vi "Export Routines.vi"(8 "error in (no error)":errorcluster, 10 "GUID":string, 11 "Section Ref in":T4 format="%.0x") -> (0 "error out":errorcluster, 1 "Routines":T1 {"Stop.Resp"."Signals"."Byte Order" items=["Little Endian", "Big Endian"]; "Stop.Resp"."Signals"."Data Type" items=["Signed", "Unsigned", "IEEE Float"]; "Stop.Cmd"."Signals"."Byte Order" items=["Little Endian", "Big Endian"]; "Stop.Cmd"."Signals"."Data Type" items=["Signed", "Unsigned", "IEEE Float"]; "Request.Resp"."Signals"."Byte Order" items=["Little Endian", "Big Endian"]; "Request.Resp"."Signals"."Data Type" items=["Signed", "Unsigned", "IEEE Float"]; "Request.Cmd"."Signals"."Byte Order" items=["Little Endian", "Big Endian"]; "Request.Cmd"."Signals"."Data Type" items=["Signed", "Unsigned", "IEEE Float"]; "Start.Resp"."Signals"."Byte Order" items=["Little Endian", "Big Endian"]; "Start.Resp"."Signals"."Data Type" items=["Signed", "Unsigned", "IEEE Float"]; "Start.Cmd"."Signals"."Byte Order" items=["Little Endian", "Big Endian"]; "Start.Cmd"."Signals"."Data Type" items=["Signed", "Unsigned", "IEEE Float"]}, 2 "Routine Refs":T5 {"Stop.Resp"."Signal Refs" format="%.0x"; "Stop.Cmd"."Signal Refs" format="%.0x"; "Status.Resp"."Signal Refs" format="%.0x"; "Status.Cmd"."Signal Refs" format="%.0x"; "Start.Resp"."Signal Refs" format="%.0x"; "Start.Cmd"."Signal Refs" format="%.0x"}, 3 "Section Ref out":T4 format="%.0x")   [LabVIEW 2015, in "Diagnostics Addon System Explorer.lvlib"]
uses:
  Diagnostics Addon System Explorer.lvlib
  <vilib>/NI Veristand/Custom Device API/Custom Device Item Ref.ctl
  Types/Routine VS References.ctl
  Types/Frame Signal VS References.ctl
  Shared/Types/Common Routines.ctl
  Shared/Types/Common Frame Parameters.ctl
  Shared/Types/Signal Parameters.ctl
  Types/FG Action.ctl
  Signal Parameters FG.vi
  <vilib>/NI Veristand/Custom Device API/NI VeriStand - Get Custom Device Channel Data.vi
  <vilib>/NI Veristand/Custom Device API/NI VeriStand - Get Item Description.vi
  <vilib>/NI Veristand/Custom Device API/NI VeriStand - Get Item Property.vi
  <vilib>/NI Veristand/Custom Device API/Get Item Property (String).vi
  <vilib>/NI Veristand/Custom Device API/Get Item Property (Double).vi
  <vilib>/NI Veristand/Custom Device API/Get Item Property (U32).vi
  <vilib>/NI Veristand/Custom Device API/NI VeriStand - Set Item Property.vi
  <vilib>/NI Veristand/Custom Device API/Set Item Property (String).vi
  <vilib>/NI Veristand/Custom Device API/Set Item Property (Double).vi
  <vilib>/NI Veristand/Custom Device API/Set Item Property (U32).vi
  Shared/SubVIs/GUID Lookup.vi
  <vilib>/NI Veristand/Custom Device Tools/Custom Device Utility Library/NI VeriStand - Search for Item by GUID.vi
  <vilib>/NI Veristand/Custom Device Tools/Custom Device Utility Library/Custom Device Utility Library.lvlib
  <vilib>/NI Veristand/Custom Device API/Custom Device API.lvlib
  Shared/Diagnostics Addon Shared.lvlib
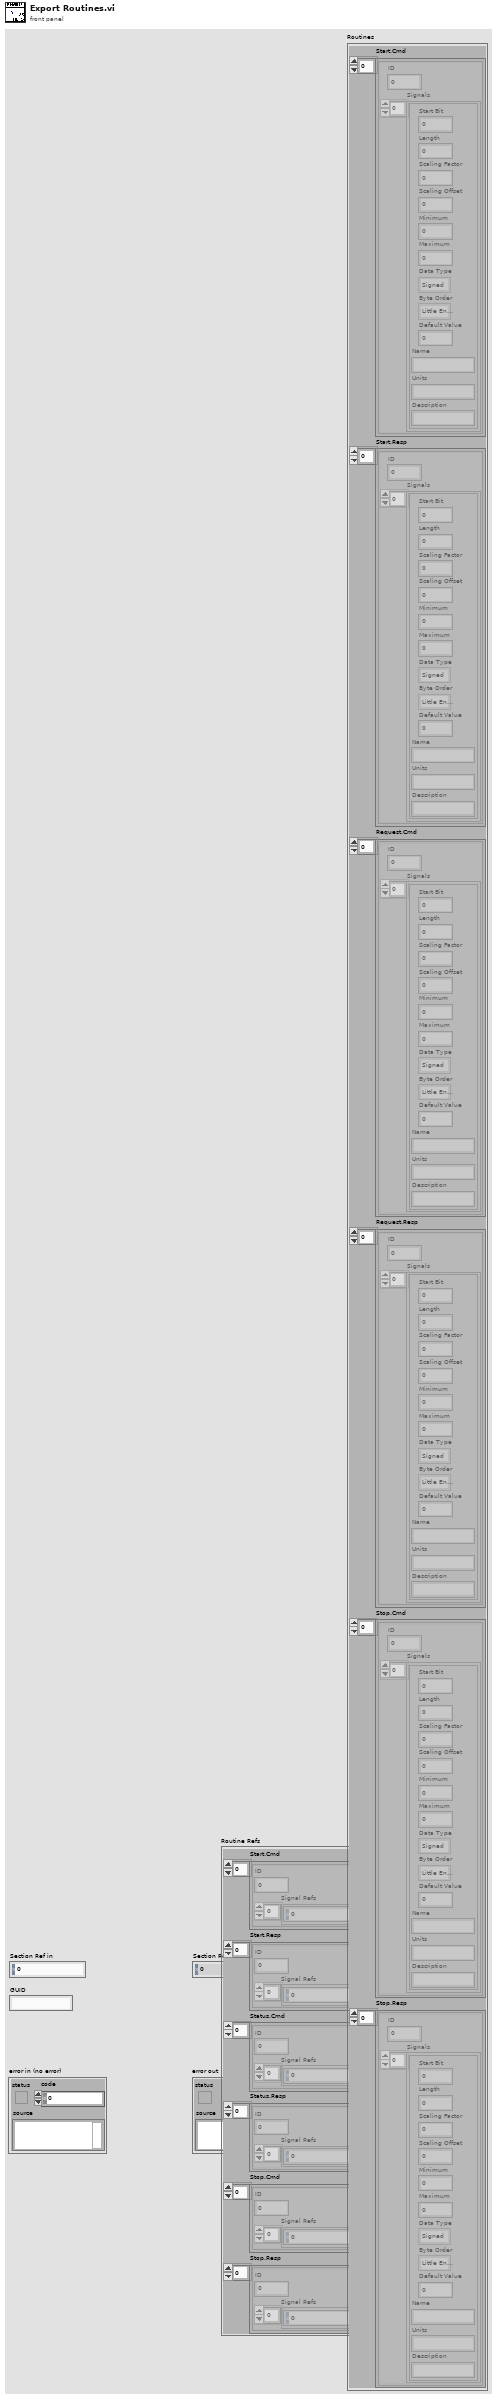
[diagram p1: front panel]
types:
  T1 = typedef "Common Routines.ctl" = cluster{"Start.Cmd":T2[], "Start.Resp":T2[], "Request.Cmd":T2[], "Request.Resp":T2[], "Stop.Cmd":T2[], "Stop.Resp":T2[]}
  T2 = typedef "Diagnostics Addon Shared.lvlib/Common Frame Parameters.ctl" = cluster{"ID":u32, "Signals":T3[]}
  T3 = typedef "Diagnostics Addon Shared.lvlib/Signal Parameters.ctl" = cluster{"Start Bit":u8, "Length":u8, "Scaling Factor":dbl, "Scaling Offset":dbl, "Minimum":dbl, "Maximum":dbl, "Data Type":u32, "Byte Order":u32, "Default Value":dbl, "Name":string, "Units":string, "Description":string}
  T4 = typedef "Custom Device API.lvlib/Custom Device Item Ref.ctl" = u64
  T5 = typedef "Diagnostics Addon System Explorer.lvlib/Routine VS References.ctl" = cluster{"Start.Cmd":T6[], "Start.Resp":T6[], "Status.Cmd":T6[], "Status.Resp":T6[], "Stop.Cmd":T6[], "Stop.Resp":T6[]}
  T6 = typedef "Diagnostics Addon System Explorer.lvlib/Frame Signal VS References.ctl" = cluster{"ID":u32, "Signal Refs":T4[]}
  T7 = typedef "Diagnostics Addon System Explorer.lvlib/FG Action.ctl" = enum16{"Get", "Set"}
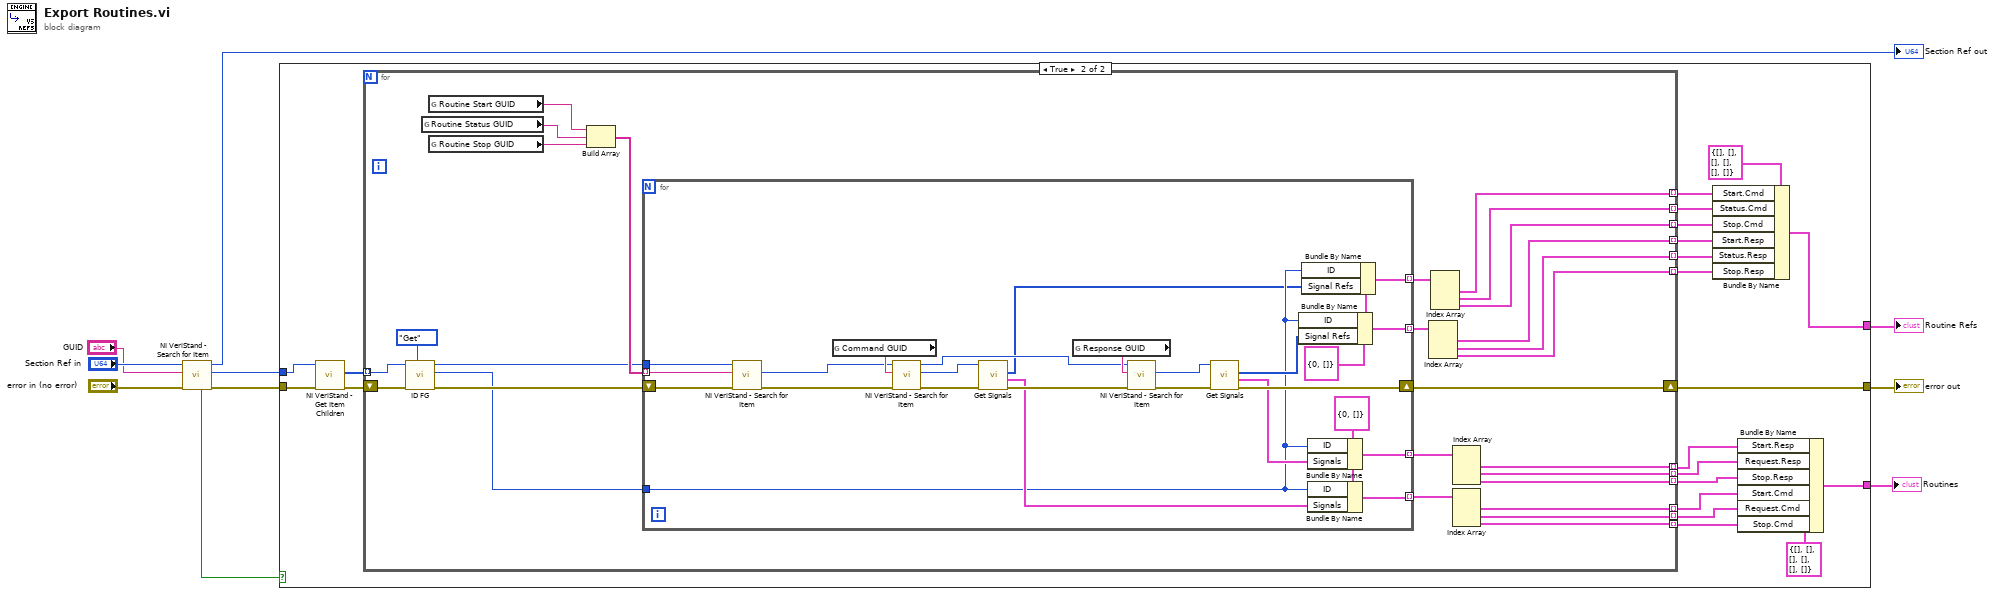
[diagram p0: block diagram]
diagram:
  n1 = call-poly <vilib>:"NI VeriStand - Search for Item.vi"("error in"="error in (no error)", "Item GUID"="GUID", "Section Ref in"="Section Ref in") -> ("error out"=w4:errorcluster, "Item Ref"=w5:T4, "Section Ref out"=→"Section Ref out":T4, "Found"=w2:bool)  [unwired: 5 in]
  n2 = case shown="True" w2 {
    tunnel: [w11 w32] -> w9
    tunnel: [_ w12] -> w8
    tunnel: w5 -> [_ w29]
    tunnel: w4 -> [w11 w28]
    tunnel: [_ w20] -> w1
    frame False {
    }
    frame True {
      n3 = call <vilib>:"NI VeriStand - Get Item Children.vi"("error in (no error)"=w28, "Item Ref in"=w29) -> ("error out"=w30:errorcluster, "Child Refs"=w31:T4[])  [unwired: 6 in, 2 out]
      n4 = for {
        shift-right: [w48] -> w32
        shift-left: w30 -> [w58]
        tunnel: w31 -> [w57] mode=indexing
        tunnel: [w46] -> w26 mode=indexing
        tunnel: [w45] -> w25 mode=indexing
        tunnel: [w44] -> w24 mode=indexing
        tunnel: [w42] -> w23 mode=indexing
        tunnel: [w41] -> w22 mode=indexing
        tunnel: [w40] -> w21 mode=indexing
        tunnel: [w38] -> w18 mode=indexing
        tunnel: [w37] -> w17 mode=indexing
        tunnel: [w36] -> w16 mode=indexing
        tunnel: [w35] -> w15 mode=indexing
        tunnel: [w34] -> w14 mode=indexing
        tunnel: [w33] -> w13 mode=indexing
        n5 = call "ID FG.vi"("Action"=FG_Action."Get", "error in (no error)"=w58, "Device Item Ref in"=w57) -> ("error out"=w51:errorcluster, "ID"=w50:u32, "Device Item Ref out"=w52:T4)  [unwired: 6 in]
        n6 = global read "GUID Lookup.vi" "Routine Status GUID"() -> (w54:string)
        n7 = global read "GUID Lookup.vi" "Routine Start GUID"() -> (w56:string)
        n8 = global read "GUID Lookup.vi" "Routine Stop GUID"() -> (w53:string)
        n9 = Build Array(w56, w54, w53) -> (w55:string[])
        n10 = for {
          tunnel: w55 -> [w84] mode=indexing
          tunnel: w52 -> [w73]
          shift-right: [w71] -> w48
          shift-left: w51 -> [w72]
          tunnel: w50 -> [w63]
          tunnel: [w67] -> w47 mode=indexing
          tunnel: [w66] -> w43 mode=indexing
          tunnel: [w64] -> w49 mode=indexing
          tunnel: [w60] -> w39 mode=indexing
          w61 = T6 {"ID"=0, "Signal Refs"=[]} ("Status.Cmd")
          w70 = T2 {"ID"=0, "Signals"=[]} ("PID In")
          n11 = call-poly <vilib>:"NI VeriStand - Search for Item.vi"("error in"=w72, "Item GUID"=w84, "Section Ref in"=w73) -> ("error out"=w74:errorcluster, "Item Ref"=w75:T4)  [unwired: 5 in, 2 out]
          n12 = global read "GUID Lookup.vi" "Command GUID"() -> (w83:string)
          n13 = call-poly <vilib>:"NI VeriStand - Search for Item.vi"("error in"=w74, "Item GUID"=w83, "Section Ref in"=w75) -> ("error out"=w80:errorcluster, "Item Ref"=w79:T4, "Section Ref out"=w81:T4)  [unwired: 5 in, 1 out]
          n14 = call "Get Signals.vi"("error in (no error)"=w80, "Device Item Ref out"=w79) -> ("error out"=w76:errorcluster, "Parameters"=w69:T3[], "Child Refs"=w62:T4[])  [unwired: 6 in, 1 out]
          n15 = global read "GUID Lookup.vi" "Response GUID"() -> (w82:string)
          n16 = call-poly <vilib>:"NI VeriStand - Search for Item.vi"("error in"=w76, "Item GUID"=w82, "Section Ref in"=w81) -> ("error out"=w78:errorcluster, "Item Ref"=w77:T4)  [unwired: 5 in, 2 out]
          n17 = call "Get Signals.vi"("error in (no error)"=w78, "Device Item Ref out"=w77) -> ("error out"=w71:errorcluster, "Parameters"=w68:T3[], "Child Refs"=w65:T4[])  [unwired: 6 in, 1 out]
          n18 = Bundle By Name(cluster=w61, "ID"=w63, "Signal Refs"=w65) -> (w64:T6)
          n19 = Bundle By Name(cluster=w61, "ID"=w63, "Signal Refs"=w62) -> (w60:T6)
          n20 = Bundle By Name(cluster=w70, "ID"=w63, "Signals"=w68) -> (w67:T2)
          n21 = Bundle By Name(cluster=w70, "ID"=w63, "Signals"=w69) -> (w66:T2)
        }
        n22 = Index Array(array=w49) -> (element #1=w35:T6, element #2=w34:T6, element #3=w33:T6)  [unwired: 3 in]
        n23 = Index Array(array=w39) -> (element #1=w38:T6, element #2=w37:T6, element #3=w36:T6)  [unwired: 3 in]
        n24 = Index Array(array=w47) -> (element #1=w46:T2, element #2=w45:T2, element #3=w44:T2)  [unwired: 3 in]
        n25 = Index Array(array=w43) -> (element #1=w42:T2, element #2=w41:T2, element #3=w40:T2)  [unwired: 3 in]
      }
      n26 = Bundle By Name(cluster=T5 {"Start.Cmd"=[], "Start.Resp"=[], "Status.Cmd"=[], "Status.Resp"=[], "Stop.Cmd"=[], "Stop.Resp"=[]} ("DIDPID Signal VS Refs"), "Start.Cmd"=w18, "Status.Cmd"=w17, "Stop.Cmd"=w16, "Start.Resp"=w15, "Status.Resp"=w14, "Stop.Resp"=w13) -> (w12:T5)
      n27 = Bundle By Name(cluster=T1 {"Start.Cmd"=[], "Start.Resp"=[], "Request.Cmd"=[], "Request.Resp"=[], "Stop.Cmd"=[], "Stop.Resp"=[]} ("Routines"), "Start.Resp"=w26, "Request.Resp"=w25, "Stop.Resp"=w24, "Start.Cmd"=w23, "Request.Cmd"=w22, "Stop.Cmd"=w21) -> (w20:T1)
    }
  }
  "error out" <- w9
  "Routine Refs" <- w8
  "Routines" <- w1
